vi "uc480_SubVI_Example_SyncEventLoop.vi"(8 "Error In":errorcluster, 10 "use sync":bool, 11 ".NET (Reference)":refnum<k24>) -> (0 "Error Out":errorcluster, 3 "Synchronize (ms)":dbl)   [LabVIEW 2016]
uses:
  C:/Users/Anatec i3/Desktop/Labview Projects/IR OPO Controller/Branches/XPS version/uc480DotNet.dll
  uc480DotNet.dll
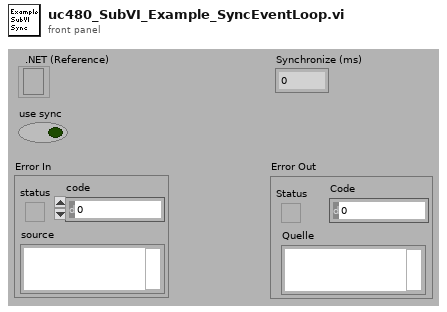
[diagram p1: front panel]
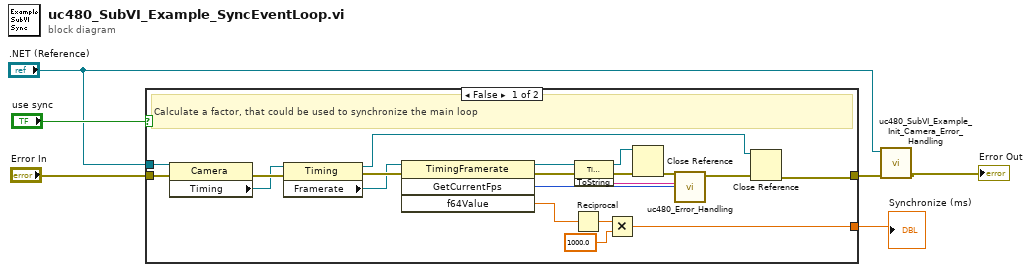
[diagram p0: block diagram]
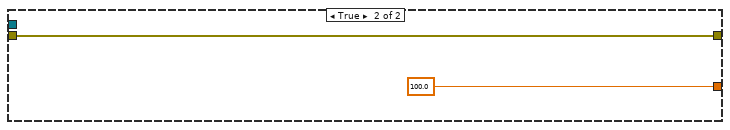
[diagram p2: hidden frame]
diagram:
  n1 = case shown="False" "use sync" {
    tunnel: [w20 100.0] -> w6
    tunnel: ".NET (Reference)" -> [w19 _]
    tunnel: "Error In" -> [w18 w28]
    tunnel: [w9 w28] -> w3
    frame False {
      # "Calculate a factor, that could be used to synchronize the main loop"
      n2 = property class="Camera"(reference=w19, error in=w18) -> (error out=w22:errorcluster, "Timing"=w21:refnum<k24>)  [unwired: 1 out]
      n3 = property class="Timing"(reference=w21, error in=w22) -> (reference out=w8:refnum<k24>, error out=w24:errorcluster, "Framerate"=w7:refnum<k24>)
      n4 = invoke class="TimingFramerate" method="GetCurrentFps"(reference=w7, error in=w24) -> (reference out=w14:refnum<k24>, error out=w15:errorcluster, "GetCurrentFps"=w16:i32, "f64Value"=w23:dbl)  [unwired: 2 in]
      n5 = Reciprocal(x=w23) -> (1/x=w26:dbl)
      n6 = invoke class="TimingFramerate" method="ToString"(reference=w14, error in=w15) -> (reference out=w13:refnum<k24>, error out=w12:errorcluster, "ToString"=w17:string)  [unwired: 1 in]
      n7 = Multiply(x=w26, y=1000.0) -> (x*y=w20:dbl)
      n8 = Close Reference(reference=w13, error in (no error)=w12) -> (error out=w11:errorcluster)
      n9 = call "uc480_Error_Handling.vi"("Error Code"=w16, "Error String"=w17, "Error In"=w11) -> ("Error Out"=w10:errorcluster)  [unwired: 8 in]
      n10 = Close Reference(reference=w8, error in (no error)=w10) -> (error out=w9:errorcluster)
    }
    frame True {
    }
  }
  "Synchronize (ms)" <- w6
  n11 = call "uc480_SubVI_Example_Init_Camera_Error_Handling.vi"("Error In"=w3, ".NET (Reference)"=".NET (Reference)") -> ("Error Out"=→"Error Out":errorcluster)  [unwired: 9 in]
